vi "Divide Polynomials.vi"   [LabVIEW 2024, in "NI_AALPro.lvlib"]
doc: "<p>Divides polynomial <strong>P(x)</strong> by polynomial <strong>Q(x)</strong>. The data types you wire to the <strong>P(x)</strong> and <strong>Q(x)</strong> inputs determine the polymorphic instance to use.</p>"
uses:
  NI_AALPro.lvlib
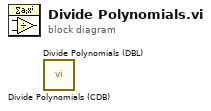
[diagram p0: block diagram]
diagram:
  n1 = call "Divide Polynomials (CDB).vi"() -> ()  [unwired: 9 in, 3 out]
  n2 = call "Divide Polynomials (DBL).vi"() -> ()  [unwired: 9 in, 3 out]
